vi "Read Button.vi"(8 "error in (no error)":errorcluster, 11 "ControlDropMsg in":refnum<class "ControlDropMsg.lvclass">) -> (0 "error out":errorcluster, 2 "Button":u16, 3 "ControlDropMsg out":refnum<class "ControlDropMsg.lvclass">)   [LabVIEW 2017, in "ActorEvents.lvlib" / "ControlDropMsg.lvclass"]
uses:
  <vilib>/gpm_packages/@cs/mva-viewable/Source/ActorEvents/IEventAggregator Messages/ControlDropMsg/ControlDropMsg.lvclass
  <vilib>/gpm_packages/@cs/mva-viewable/Source/ActorEvents/IEventAggregator Messages/ControlDropMsg/ControlDropMsg.lvclass/ControlDropMsg.ctl
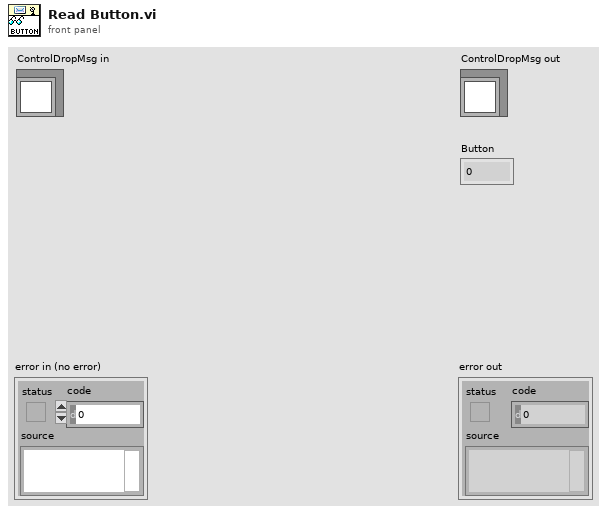
[diagram p1: front panel]
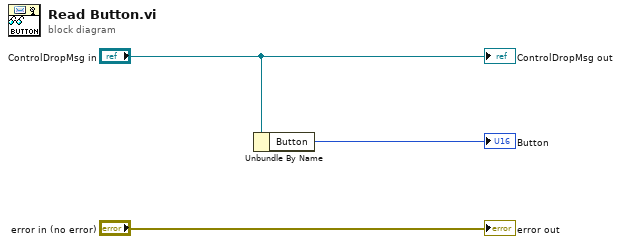
[diagram p0: block diagram]
diagram:
  n1 = Unbundle By Name("ControlDropMsg in") -> ("Button"=→"Button":u16)
  "error out" <- "error in (no error)"
  "ControlDropMsg out" <- "ControlDropMsg in"
